vi "Relocation.vi"() -> ()   [LabVIEW 2014]
uses:
  <vilib>/Instr/_visa.llb/VISA Configure Serial Port (Instr).vi
panel:
  out "ERROut?":string
  in  "Destination length um":dbl
  in  "Step length um":dbl
  in  "Withdraw a step":bool
  in  "Move a step towards":bool
  in  "Move to":bool
  out "RoughZPosDia":dbl(graph)
  in  "Confirm":bool
  out "RoughZPos um":dbl
  out "ERRIn?":string
  in  "RoughXYZ":refnum<visa-resource-name>
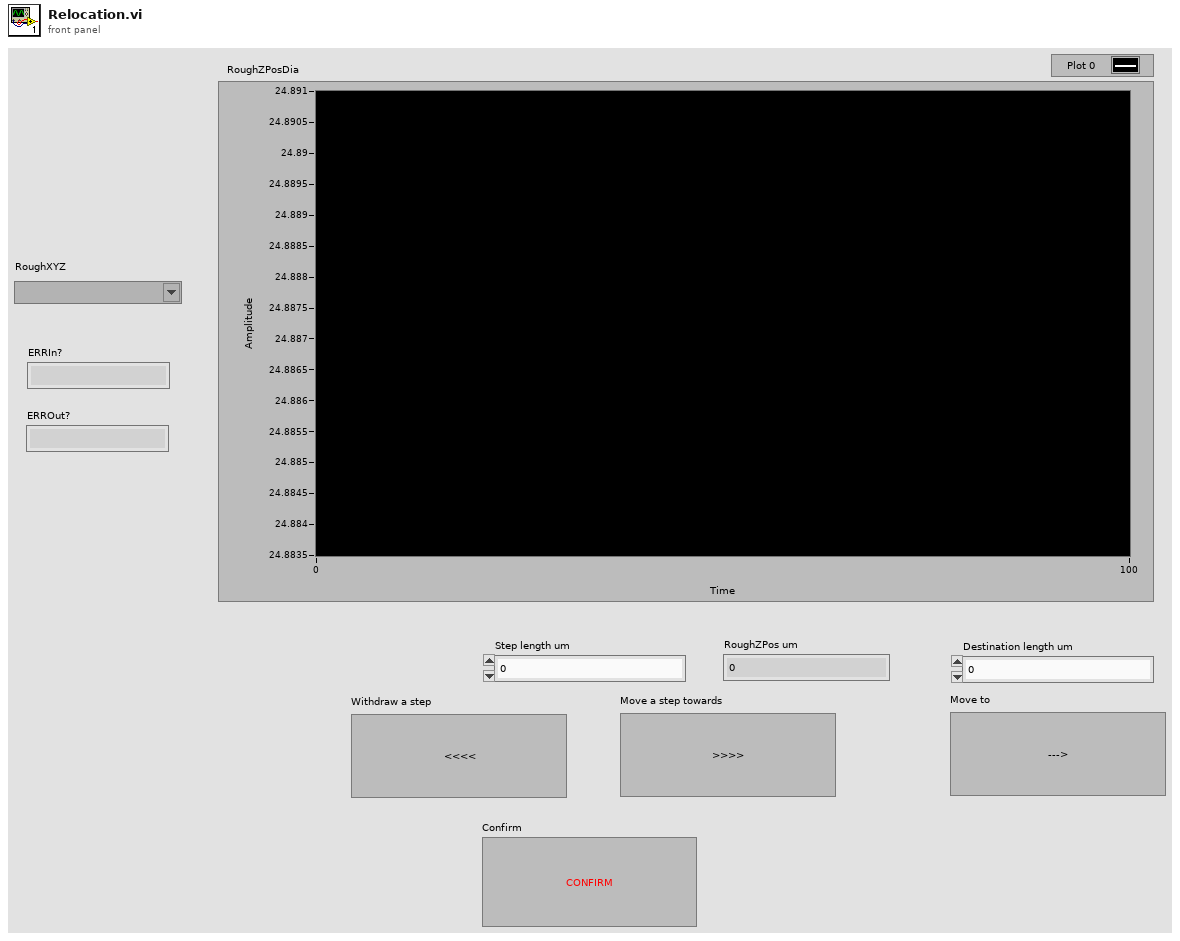
[diagram p1: front panel]
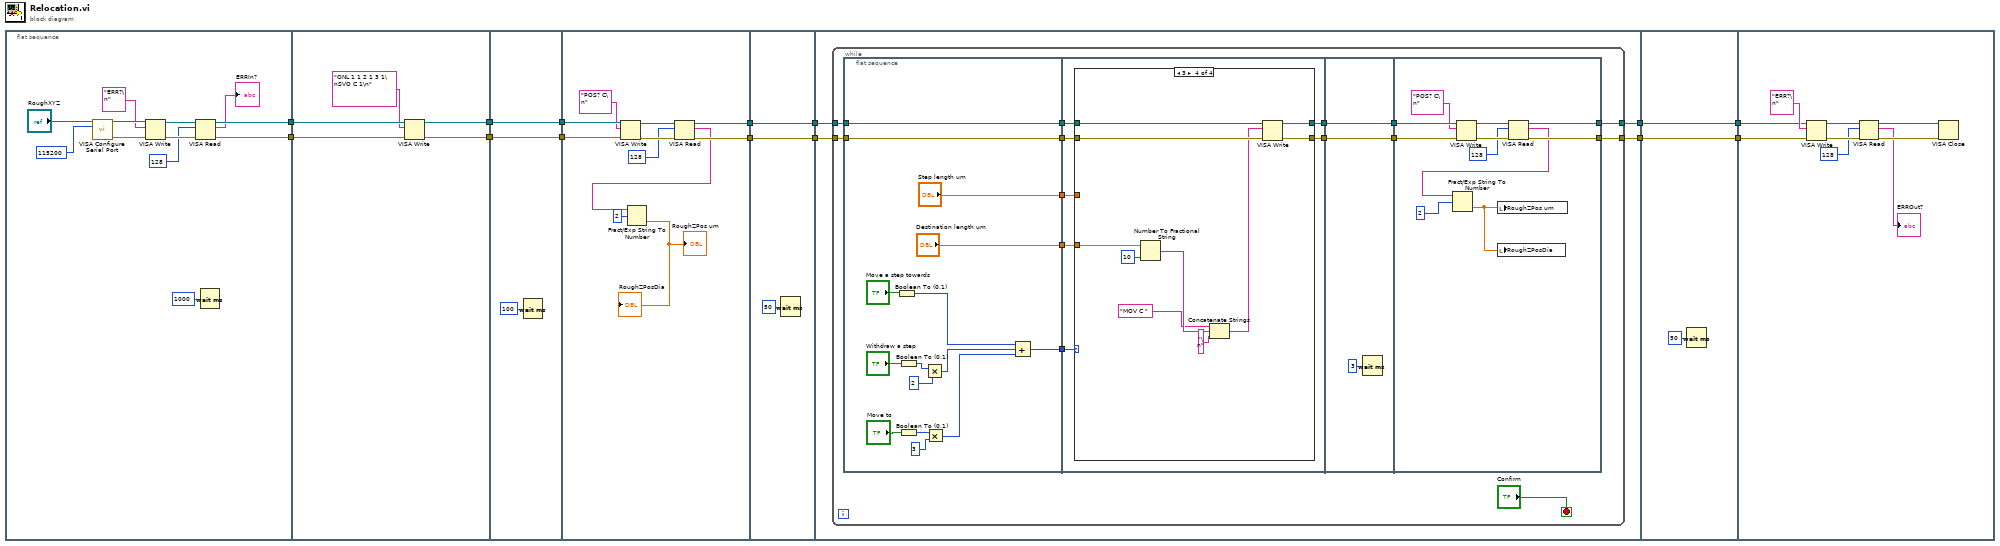
[diagram p0: block diagram]
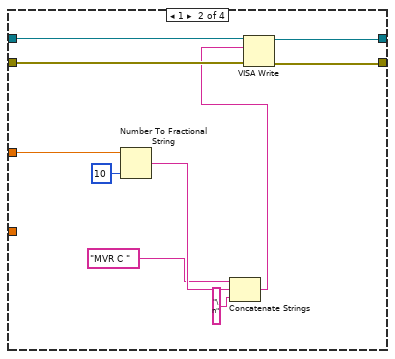
[diagram p3: hidden frame]
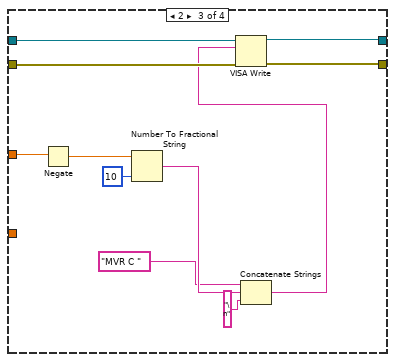
[diagram p4: hidden frame]
diagram:
  n1 = flat-sequence {
    tunnel: [w18] -> w14
    tunnel: [w17] -> w13
    tunnel: w14 -> [w31]
    tunnel: w13 -> [w30]
    tunnel: [w28] -> w12
    tunnel: [w27] -> w11
    tunnel: w12 -> [w33]
    tunnel: w11 -> [w32]
    tunnel: [w33] -> w10
    tunnel: [w32] -> w9
    tunnel: w10 -> [w45]
    tunnel: w9 -> [w44]
    tunnel: [w39] -> w8
    tunnel: [w38] -> w7
    tunnel: w8 -> [w47]
    tunnel: w7 -> [w46]
    tunnel: [w47] -> w6
    tunnel: [w46] -> w5
    tunnel: w6 -> [w52]
    tunnel: w5 -> [w51]
    tunnel: [w50] -> w4
    tunnel: [w49] -> w3
    tunnel: w4 -> [w137]
    tunnel: w3 -> [w136]
    tunnel: [w137] -> w2
    tunnel: [w136] -> w1
    tunnel: w2 -> [w143]
    tunnel: w1 -> [w142]
    frame #0 {
      n2 = call-poly "VISA Configure Serial Port"("VISA resource name"="RoughXYZ", "baud rate (9600)"=u32 115200) -> ("VISA resource name out"=w24:refnum<visa-resource-name>, "error out"=w23:errorcluster)  [unwired: 12 in]
      n3 = VISA Write(VISA resource name=w24, write buffer="ERR?\n", error in (no error)=w23) -> (VISA resource name out=w21:refnum<visa-resource-name>, error out=w20:errorcluster)  [unwired: 1 out]
      n4 = VISA Read(VISA resource name=w21, byte count=u32 128, error in (no error)=w20) -> (VISA resource name out=w18:refnum<visa-resource-name>, read buffer=→"ERRIn?":string, error out=w17:errorcluster)  [unwired: 1 out]
      n5 = Wait (ms)(milliseconds to wait=u32 1000) -> ()  [unwired: 1 out]
    }
    frame #1 {
      n6 = VISA Write(VISA resource name=w31, write buffer="ONL 1 1 2 1 3 1\nSVO C 1\n", error in (no error)=w30) -> (VISA resource name out=w28:refnum<visa-resource-name>, error out=w27:errorcluster)  [unwired: 1 out]
    }
    frame #2 {
      n7 = Wait (ms)(milliseconds to wait=u32 100) -> ()  [unwired: 1 out]
    }
    frame #3 {
      n8 = VISA Write(VISA resource name=w45, write buffer="POS? C\n", error in (no error)=w44) -> (VISA resource name out=w42:refnum<visa-resource-name>, error out=w41:errorcluster)  [unwired: 1 out]
      n9 = VISA Read(VISA resource name=w42, byte count=u32 128, error in (no error)=w41) -> (VISA resource name out=w39:refnum<visa-resource-name>, read buffer=w37:string, error out=w38:errorcluster)  [unwired: 1 out]
      n10 = Fract/Exp String To Number(string=w37, offset=2) -> (number=→"RoughZPos um" →"RoughZPosDia":dbl)  [unwired: 2 in, 1 out]
    }
    frame #4 {
      n11 = Wait (ms)(milliseconds to wait=u32 50) -> ()  [unwired: 1 out]
    }
    frame #5 {
      n12 = while {
        tunnel: w52 -> [w65]
        tunnel: w51 -> [w64]
        tunnel: [w54] -> w50
        tunnel: [w53] -> w49
        stop <- "Confirm" stop-if-true
        n13 = flat-sequence {
          tunnel: w65 -> [w81]
          tunnel: w64 -> [w80]
          tunnel: [w81] -> w63
          tunnel: [w80] -> w62
          tunnel: [w69] -> w61
          tunnel: ["Step length um"] -> w58
          tunnel: ["Destination length um"] -> w57
          tunnel: w63 -> [w88]
          tunnel: w62 -> [w87]
          tunnel: w61 -> [w86]
          tunnel: [w85] -> w60
          tunnel: [w84] -> w59
          tunnel: w58 -> [w83]
          tunnel: w57 -> [w82]
          tunnel: w60 -> [w123]
          tunnel: w59 -> [w122]
          tunnel: [w123] -> w56
          tunnel: [w122] -> w55
          tunnel: w56 -> [w135]
          tunnel: w55 -> [w134]
          tunnel: [w129] -> w54
          tunnel: [w128] -> w53
          frame #0 {
            n14 = Boolean To (0,1)(Boolean="Move a step towards") -> (0, 1=w72:i16)
            n15 = Boolean To (0,1)(Boolean="Withdraw a step") -> (0, 1=w76:i16)
            n16 = Boolean To (0,1)(Boolean="Move to") -> (0, 1=w74:i16)
            n17 = Multiply(x=w76, y=i16 2) -> (x*y=w71:i16)
            n18 = Multiply(x=w74, y=i16 3) -> (x*y=w70:i16)
            n19 = Compound Arithmetic op=ADD(w72, w71, w70) -> (w69:i16)
          }
          frame #1 {
            n20 = case shown="3" w86 {
              tunnel: w88 -> [w90 w95 w103 w119]
              tunnel: w87 -> [w89 w94 w102 w118]
              tunnel: [w90 w93 w105 w121] -> w85
              tunnel: [w89 w92 w104 w120] -> w84
              tunnel: w83 -> [_ w100 w107 _]
              tunnel: w82 -> [_ _ _ w113]
              frame 0, Default {
              }
              frame 1 {
                n21 = Number To Fractional String(number=w100, precision (6)=i16 10) -> (F-format string=w98:string)  [unwired: 2 in]
                n22 = Concatenate Strings("MVR C " ("string"), w98, "\n" ("string")) -> (w91:string)
                n23 = VISA Write(VISA resource name=w95, write buffer=w91, error in (no error)=w94) -> (VISA resource name out=w93:refnum<visa-resource-name>, error out=w92:errorcluster)  [unwired: 1 out]
              }
              frame 2 {
                n24 = Negate(x=w107) -> (-x=w106:dbl)
                n25 = Number To Fractional String(number=w106, precision (6)=i16 10) -> (F-format string=w110:string)  [unwired: 2 in]
                n26 = Concatenate Strings("MVR C " ("string"), w110, "\n" ("string")) -> (w101:string)
                n27 = VISA Write(VISA resource name=w103, write buffer=w101, error in (no error)=w102) -> (VISA resource name out=w105:refnum<visa-resource-name>, error out=w104:errorcluster)  [unwired: 1 out]
              }
              frame 3 {
                n28 = Number To Fractional String(number=w113, precision (6)=i16 10) -> (F-format string=w116:string)  [unwired: 2 in]
                n29 = Concatenate Strings("MOV C " ("string"), w116, "\n" ("string")) -> (w112:string)
                n30 = VISA Write(VISA resource name=w119, write buffer=w112, error in (no error)=w118) -> (VISA resource name out=w121:refnum<visa-resource-name>, error out=w120:errorcluster)  [unwired: 1 out]
              }
            }
          }
          frame #2 {
            n31 = Wait (ms)(milliseconds to wait=u32 3) -> ()  [unwired: 1 out]
          }
          frame #3 {
            n32 = VISA Write(VISA resource name=w135, write buffer="POS? C\n", error in (no error)=w134) -> (VISA resource name out=w132:refnum<visa-resource-name>, error out=w131:errorcluster)  [unwired: 1 out]
            n33 = VISA Read(VISA resource name=w132, byte count=u32 128, error in (no error)=w131) -> (VISA resource name out=w129:refnum<visa-resource-name>, read buffer=w127:string, error out=w128:errorcluster)  [unwired: 1 out]
            n34 = Fract/Exp String To Number(string=w127, offset=2) -> (number=w125:dbl)  [unwired: 2 in, 1 out]
            n35 = local write "RoughZPos um"(w125) -> ()
            n36 = local write "RoughZPosDia"(w125) -> ()
          }
        }
      }
    }
    frame #6 {
      n37 = Wait (ms)(milliseconds to wait=u32 50) -> ()  [unwired: 1 out]
    }
    frame #7 {
      n38 = VISA Write(VISA resource name=w143, write buffer="ERR?\n", error in (no error)=w142) -> (VISA resource name out=w146:refnum<visa-resource-name>, error out=w145:errorcluster)  [unwired: 1 out]
      n39 = VISA Read(VISA resource name=w146, byte count=u32 128, error in (no error)=w145) -> (VISA resource name out=w141:refnum<visa-resource-name>, read buffer=→"ERROut?":string, error out=w140:errorcluster)  [unwired: 1 out]
      n40 = VISA Close(VISA resource name=w141, error in (no error)=w140) -> ()  [unwired: 1 out]
    }
  }
